vi "Dot Product.vi"(1 "B":sgl[](array[numeric]), 2 "A":sgl[](array[numeric])) -> (0 "c":sgl)   [LabVIEW 2020]
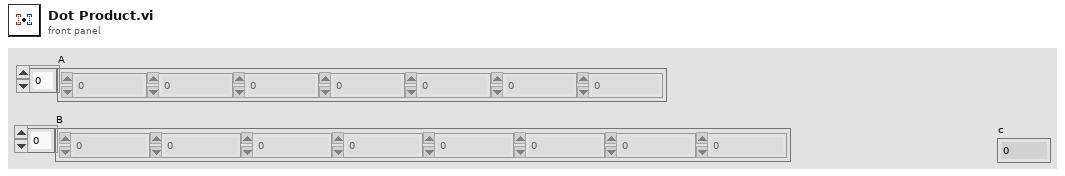
[diagram p1: front panel]
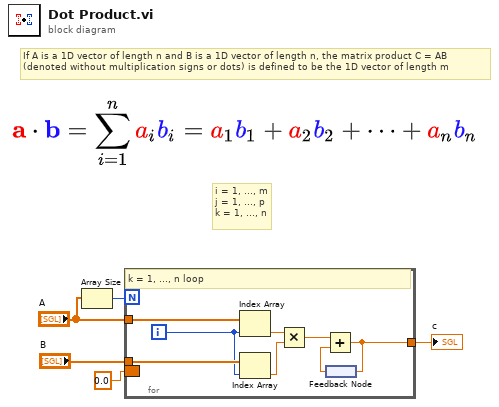
[diagram p0: block diagram]
diagram:
  # "If A is a 1D vector of length n and B is a 1D vector of length n, the matrix product C = AB \n(denoted without multiplication signs or dots) is defined to be the 1D vector of length m"
  # "i = 1, ..., m\nj = 1, ..., p\nk = 1, ..., n"
  n1 = Array Size(array="A") -> (size(s)=w1:i32)
  n2 = for {
    N: w1 -> [_]
    tunnel: "A" -> [w13]
    tunnel: "B" -> [w12]
    tunnel: [w7] -> w3
    border: sgl 0.0 -> [_]
    i -> [w6]
    # "k = 1, ..., n loop"
    n3 = Index Array(array=w13, index=w6) -> (element=w11:sgl)
    n4 = Index Array(array=w12, index=w6) -> (element=w10:sgl)
    n5 = Multiply(x=w11, y=w10) -> (x*y=w9:sgl)
    n6 = feedback #1() -> (w8:sgl)
    n7 = Add(x=w9, y=w8) -> (x+y=w7:sgl)
    n8 = feedback-in #1(w7) -> ()
  }
  "c" <- w3
